vi "Disconnect.vi"(8 "error in (no error)":errorcluster, 11 "TwinCAT ADS in":refnum<class "TwinCAT ADS.lvclass">) -> (0 "error out":errorcluster)   [LabVIEW 2018, in "TwinCAT ADS.lvclass"]
uses:
  TwinCAT ADS.lvclass
  TwinCAT ADS.lvclass/TwinCAT ADS.ctl
  TwinCAT.Ads
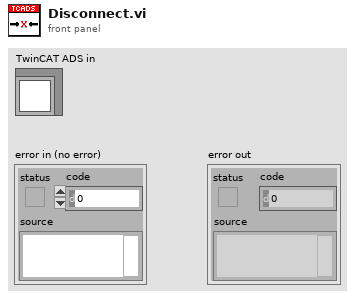
[diagram p1: front panel]
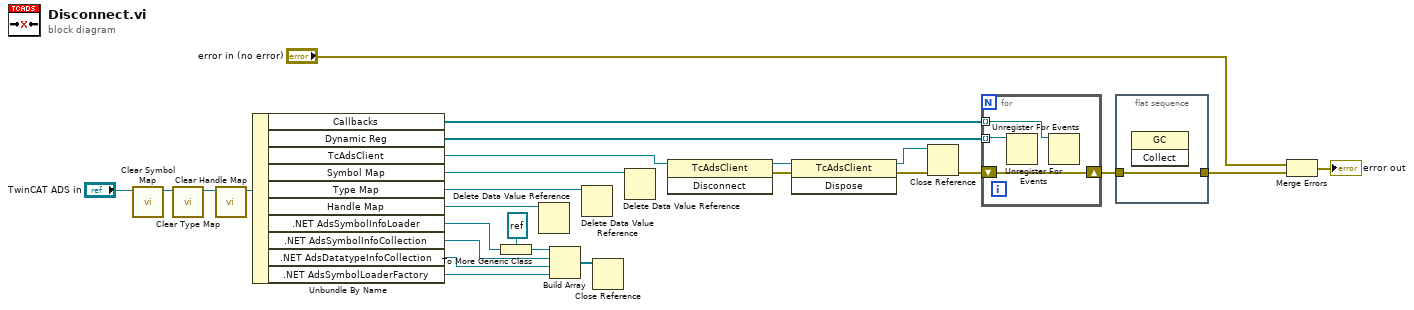
[diagram p0: block diagram]
diagram:
  n1 = call "Clear Symbol Map.vi"("TwinCAT ADS in"="TwinCAT ADS in") -> ("TwinCAT ADS out"=w4:refnum<class "TwinCAT ADS.lvclass">)  [unwired: 9 in, 1 out]
  n2 = call "Clear Type Map.vi"("TwinCAT ADS in"=w4) -> ("TwinCAT ADS out"=w3:refnum<class "TwinCAT ADS.lvclass">)  [unwired: 9 in, 1 out]
  n3 = call "Clear Handle Map.vi"("TwinCAT ADS in"=w3) -> ("TwinCAT ADS out"=w2:refnum<class "TwinCAT ADS.lvclass">)  [unwired: 9 in, 1 out]
  n4 = Unbundle By Name(w2) -> ("Callbacks"=w17:refnum<k27>[], "Dynamic Reg"=w18:refnum<event-registration>[], "TcAdsClient"=w25:refnum<k24>, "Symbol Map"=w13:refnum<data-value>, "Type Map"=w12:refnum<data-value>, "Handle Map"=w1:refnum<data-value>, ".NET AdsSymbolInfoLoader"=w11:refnum<k24>, ".NET AdsSymbolInfoCollection"=w8:refnum<k24>, ".NET AdsDatatypeInfoCollection"=w7:refnum<k24>, ".NET AdsSymbolLoaderFactory"=w6:refnum<k24>)
  n5 = To More Generic Class(target class=refnum<k24> refnum (".NET object"), reference=w11) -> (generic class reference=w10:refnum<k24>)
  n6 = Delete Data Value Reference(data value reference=w1) -> ()  [unwired: 1 in, 2 out]
  n7 = Build Array(w10, w8, w7, w6) -> (w9:refnum<k24>[])
  n8 = Delete Data Value Reference(data value reference=w12) -> ()  [unwired: 1 in, 2 out]
  n9 = Close Reference(reference=w9) -> ()  [unwired: 1 in, 1 out]
  n10 = Delete Data Value Reference(data value reference=w13) -> ()  [unwired: 1 in, 2 out]
  n11 = invoke class="TcAdsClient" method="Disconnect"(reference=w25) -> (reference out=w24:refnum<k24>, error out=w26:errorcluster)  [unwired: 2 in, 1 out]
  n12 = invoke class="TcAdsClient" method="Dispose"(reference=w24, error in=w26) -> (reference out=w22:refnum<k24>, error out=w23:errorcluster)  [unwired: 1 in, 1 out]
  n13 = Close Reference(reference=w22, error in (no error)=w23) -> (error out=w21:errorcluster)
  n14 = for {
    tunnel: w17 -> [w29] mode=indexing
    tunnel: w18 -> [w28] mode=indexing
    shift-right: [w27] -> w20
    shift-left: w21 -> [w27]
    n15 = Unregister For Events(event registration refnum=w28) -> ()  [unwired: 1 in, 1 out]
    n16 = Unregister For Events(event registration refnum=w29) -> ()  [unwired: 1 in, 1 out]
  }
  n17 = flat-sequence {
    tunnel: [w30] -> w16
    tunnel: w20 -> [w30]
    frame #0 {
      n18 = invoke class="GC" method="Collect"() -> ()  [unwired: 3 in, 3 out]
    }
  }
  n19 = Merge Errors("error in (no error)", w16) -> (→"error out":errorcluster)
